vi "Write Timestamped Array to CSV.vi"(2 "error in":errorcluster, 3 "numbers":dbl[](array[numeric]), 4 "csv file (in)":refnum<file>) -> (0 "error out":errorcluster, 1 "csv file (out)":refnum<file>)   [LabVIEW 2016]
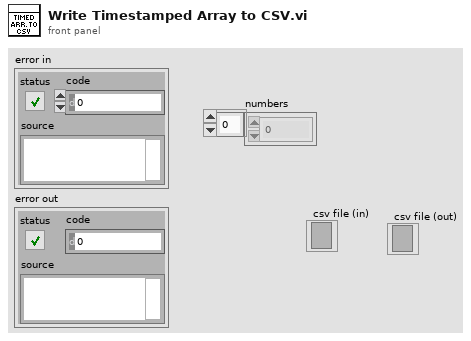
[diagram p1: front panel]
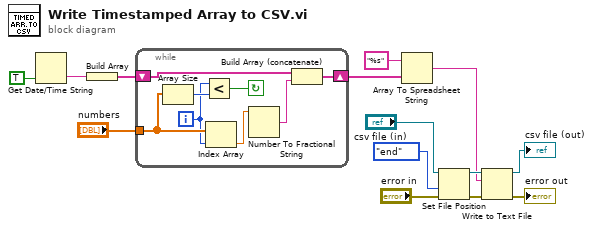
[diagram p0: block diagram]
diagram:
  n1 = Get Date/Time String(want seconds? (F)=TRUE) -> (time string=w2:string)  [unwired: 2 in, 1 out]
  n2 = Build Array(w2) -> (w3:string[])
  n3 = while {
    tunnel: "numbers" -> [w20]
    shift-right: [w15] -> w1
    shift-left: w3 -> [w17]
    i -> [w19]
    stop <- w21 continue-if-true
    n4 = Array Size(array=w20) -> (size(s)=w22:i32)
    n5 = Less?(x=w19, y=w22) -> (x < y?=w21:bool)
    n6 = Index Array(array=w20, index=w19) -> (element=w18:dbl)
    n7 = Number To Fractional String(number=w18) -> (F-format string=w16:string)  [unwired: 3 in]
    n8 = Build Array (concatenate)(w17, w16) -> (w15:string[])
  }
  n9 = Array To Spreadsheet String(array=w1, 3:"%s" ("format string")) -> (spreadsheet string=w11:string)  [unwired: 1 in]
  n10 = Set File Position(refnum="csv file (in)", from (0:start)=enum16{"start", "end", "current"}."end", error in="error in") -> (refnum out=w13:refnum<file>, error out=w7:errorcluster)  [unwired: 1 in]
  n11 = Write to Text File(file (use dialog)=w13, text=w11, error in=w7) -> (refnum out=→"csv file (out)":refnum<file>, error out=→"error out":errorcluster)  [unwired: 1 in, 1 out]
